vi "command send GPIB.vi"(3 "error in":errorcluster, 4 "Command":string, 5 "addres":string="18") -> (0 "error out":errorcluster)   [LabVIEW 2013]
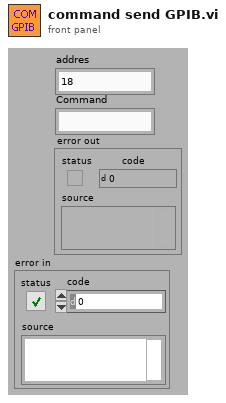
[diagram p1: front panel]
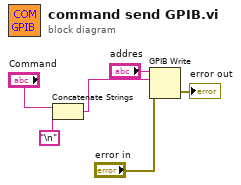
[diagram p0: block diagram]
diagram:
  n1 = Concatenate Strings("Command", "\n") -> (w4:string)
  n2 = GPIB Write(0:"addres", 1:w4, 3:"error in") -> (6:→"error out":errorcluster)  [unwired: 3 out]
